vi "neopixel control loop.vi"   [LabVIEW 2016]
uses:
  <vilib>/Platform/TimedLoop/XDataNode/timing_clust.ctl
  <vilib>/Platform/TimedLoop/XDataNode/nitl_modes.ctl
  <vilib>/Platform/TimedLoop/XDataNode/wakeup.ctl
  <vilib>/platform/TimedLoop/XDataNode/XDataNode.xnode
  <vilib>/Platform/TimedLoop/XDataNode/XDNodeRunTimeDep.lvlib
types:
  T1 = typedef "WPI_I2CDevRef.ctl" = cluster{"DevStatus":errorcluster, "Device Address":u8, "Handle":i32, "I2C Bus":T2}
  T2 = typedef "i2c_bus.ctl" = enum16{"I2C On-Board", "I2C MXP", "Invalid"}
  T3 = typedef "XDNodeRunTimeDep.lvlib/timing_clust.ctl" = cluster{"Expected End [f-1]":u64, "Actual End [f-1]":u64, "Finished Late? [f-1]":bool, "Expected End [i-1]":u64, "Actual End [i-1]":u64, "Finished Late? [i-1]":bool, "Expected Start [i]":u64, "Actual Start [i]":u64, "Expected Start [f]":u64, "Actual Start [f]":u64, "Source Name":string, "Structure Name":string, "Period":i64, "Deadline":i64, "Offset":i64, "Start":i64, "Priority":i32, "Timeout":i32, "Mode":T4, "Wakeup Reason":T5, "Error":errorcluster, "Source Type":string, "Secondary Source Type":string, "Global End Time":u64, "Global Start Time":u64, "Frame Duration":u64, "Iteration Duration":u64, "Assigned CPU":i32, "I/O Scan Engine Mode":u32}
  T4 = typedef "XDNodeRunTimeDep.lvlib/nitl_modes.ctl" = enum32{"No Change", "Process missed periods, maintain original phase", "Discard missed periods, maintain original phase", "Process missed periods, ignore original phase", "Discard missed periods, ignore original phase"}
  T5 = typedef "XDNodeRunTimeDep.lvlib/wakeup.ctl" = enum32{"Normal", "Aborted", "Asynchronous wakeup", "Timing source error", "Timed loop error", "Timeout"}
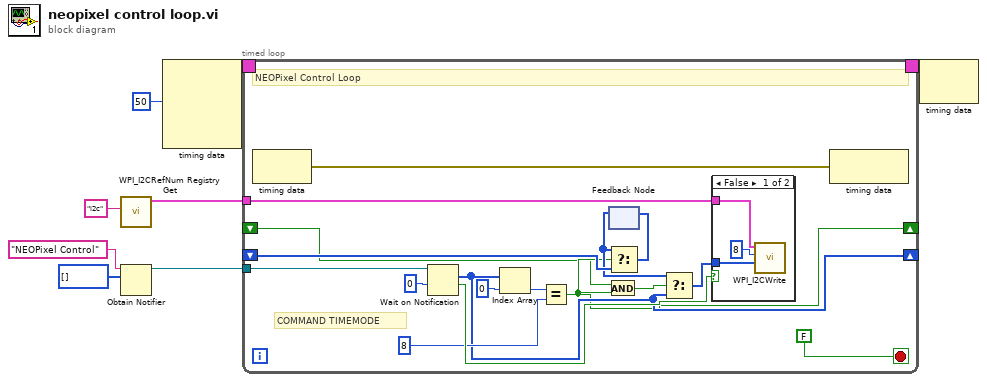
[diagram p0: block diagram]
diagram:
  n1 = call <vilib>:"WPI_I2CRefNum Registry Get.vi"("refnum name"="i2c") -> ("I2CDevRef"=w2:T1)  [unwired: 9 in, 1 out]
  n2 = Obtain Notifier(name (unnamed)="NEOPixel Control", notification data type=u8[] []) -> (notifier out=w4:refnum<notifier>)  [unwired: 2 in, 2 out]
  n3 = node-c288(i64 50 ("Period")) -> (w8:T3)  [unwired: 3 in]
  n4 = timed-loop {
    tunnel: w4 -> [w25]
    timing: w8 -> [_]
    timing-out: [_] -> w7
    tunnel: w2 -> [w22]
    shift-right: [w15] -> _
    shift-left: _ -> [w21]
    shift-right: [w13] -> _
    shift-left: _ -> [w12]
    stop <- FALSE stop-if-true
    # "COMMAND TIMEMODE"
    # "NEOPixel Control Loop"
    n5 = node-c288() -> (w16:errorcluster)  [unwired: 1 in]
    n6 = Wait on Notification(notifier=w25, timeout in ms (-1)=0) -> (notification=w15:u8[], timed out?=w23:bool)  [unwired: 2 in, 2 out]
    n7 = Index Array(array=w15, index=0) -> (element=w18:u8)
    n8 = Equal?(x=w18, y=u8 8) -> (x = y?=w13:bool)
    n9 = And(x=w12, y=w13) -> (x .and. y?=w11:bool)
    n10 = feedback #1() -> (w14:u8[])  [unwired: 1 in]
    n11 = Select(t=w14, s=w13, f=w21) -> (s? t:f=w20:u8[])
    n12 = feedback-in #1(w20) -> ()
    n13 = Select(t=w14, s=w11, f=w15) -> (s? t:f=w10:u8[])
    n14 = case shown="False" w23 {
      tunnel: w10 -> [w26 _]
      tunnel: w22 -> [w28 _]
      frame False {
        n15 = call <vilib>:"WPI_I2CWrite.vi"("I2CDataToSend"=w26, "I2CRegister"=u8 8, "I2CDevRef"=w28) -> ()  [unwired: 7 in, 2 out]
      }
      frame True {
      }
    }
    n16 = node-c288(w16) -> ()  [unwired: 1 out]
  }
  n17 = node-c288(w7) -> ()  [unwired: 1 out]
